vi "Single Cscan - DAQ Trigger.vi"(6 "Frequency":cluster{"Clock, kHz":dbl, "Freq, kHz":dbl}={"Clock, kHz"=920.0, "Freq, kHz"=46.0} {"Clock, kHz" format="%#_13g"}, 7 "# Extra":cluster{"# ARpt_extra":i32, "#Brtn_extra":i32}={"# ARpt_extra"=5, "#Brtn_extra"=40}, 9 "Galvo VPP":cluster{"VPP-X":dbl, "VPP-Y":dbl}={"VPP-X"=5.0, "VPP-Y"=5.0}, 10 "Scan Repeat":cluster{"# A rpt":i32, "# B rpt":i32}={"# A rpt"=1, "# B rpt"=1}, 11 "# Points":cluster{"# Aline":i32, "# B scan":i32}={"# Aline"=500, "# B scan"=500}) -> (2 "Galvo X&Trigger":waveform(dbl)[](graph)=[{"t0"=timestamp(0 s since 1904-01-01), "dt"=1.0, "Y"=array[3800 elements]}, {"t0"=timestamp(0 s since 1904-01-01), "dt"=1.0, "Y"=array[3800 elements]}])   [LabVIEW 2017]
uses:
  <vilib>/Waveform/WDTOps.llb/WDT Append Waveforms DBL.vi
  <vilib>/measure/NI_MABase.lvlib
panel:
  out "input cluster":cluster{"Fs":dbl, "#s":dbl}
  out "size(s)":i32
  out "#Brtn_extra":i32
  out "dVY":dbl
  out "# A Rpt Delay":i32
  out "# B rtn":i32
  out "# A repeat":i32
  out "dVX":dbl
  out "S/F":dbl
  out "VPP-Y":dbl
  out "VPP-X":dbl
  out "Clock, kHz":dbl
  out "Freq, kHz":dbl
  out "# A Total":i32
  out "# Aline":i32
  out "# B scan":i32
  out "# B Repeat":i32
  # "Single Cscan - DAQ Trigger"
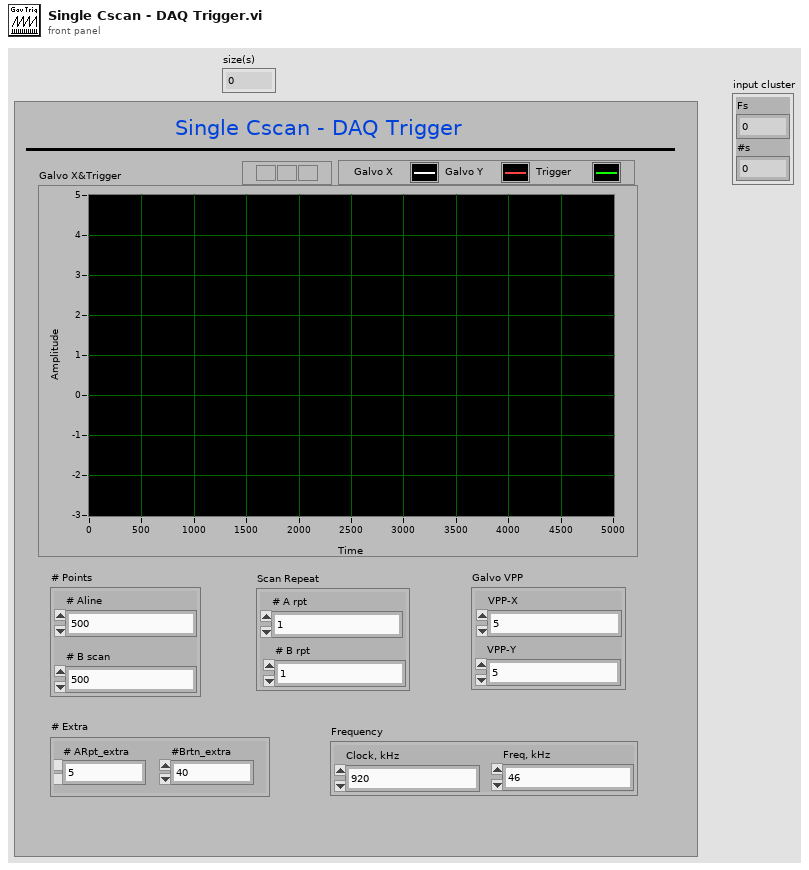
[diagram p1: front panel]
types:
  T1 = enum16{"Sine Wave", "Triangle Wave", "Square Wave", "Sawtooth Wave"}
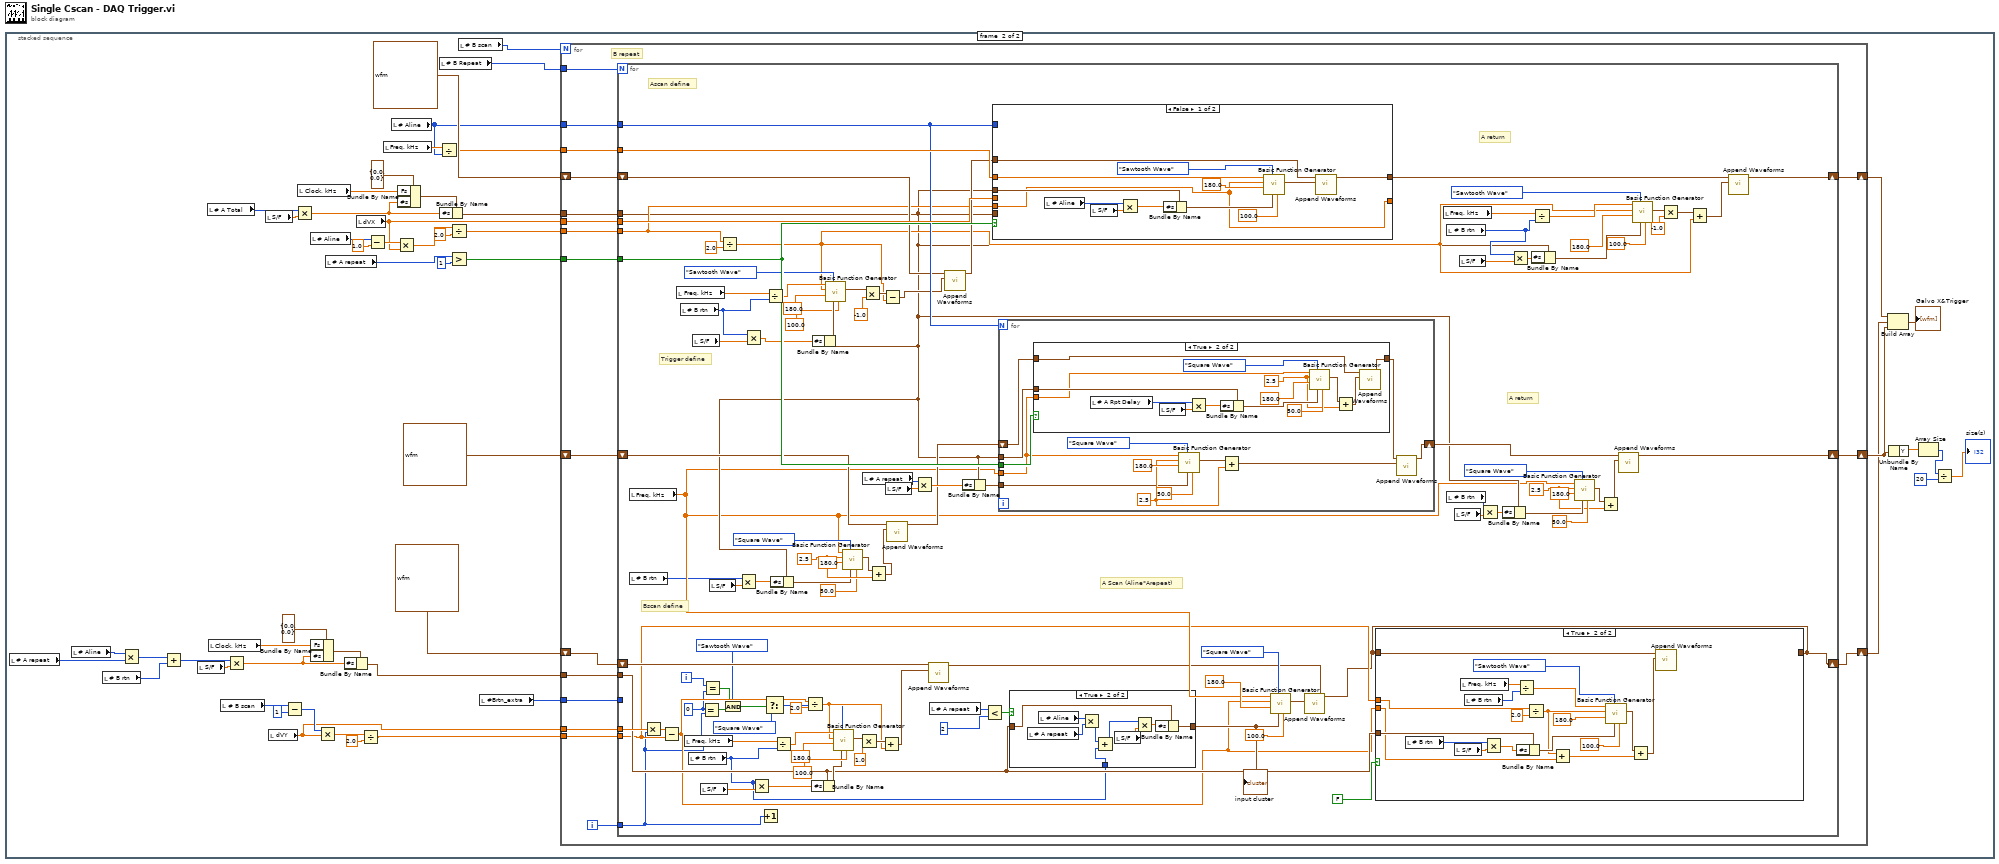
[diagram p0: block diagram]
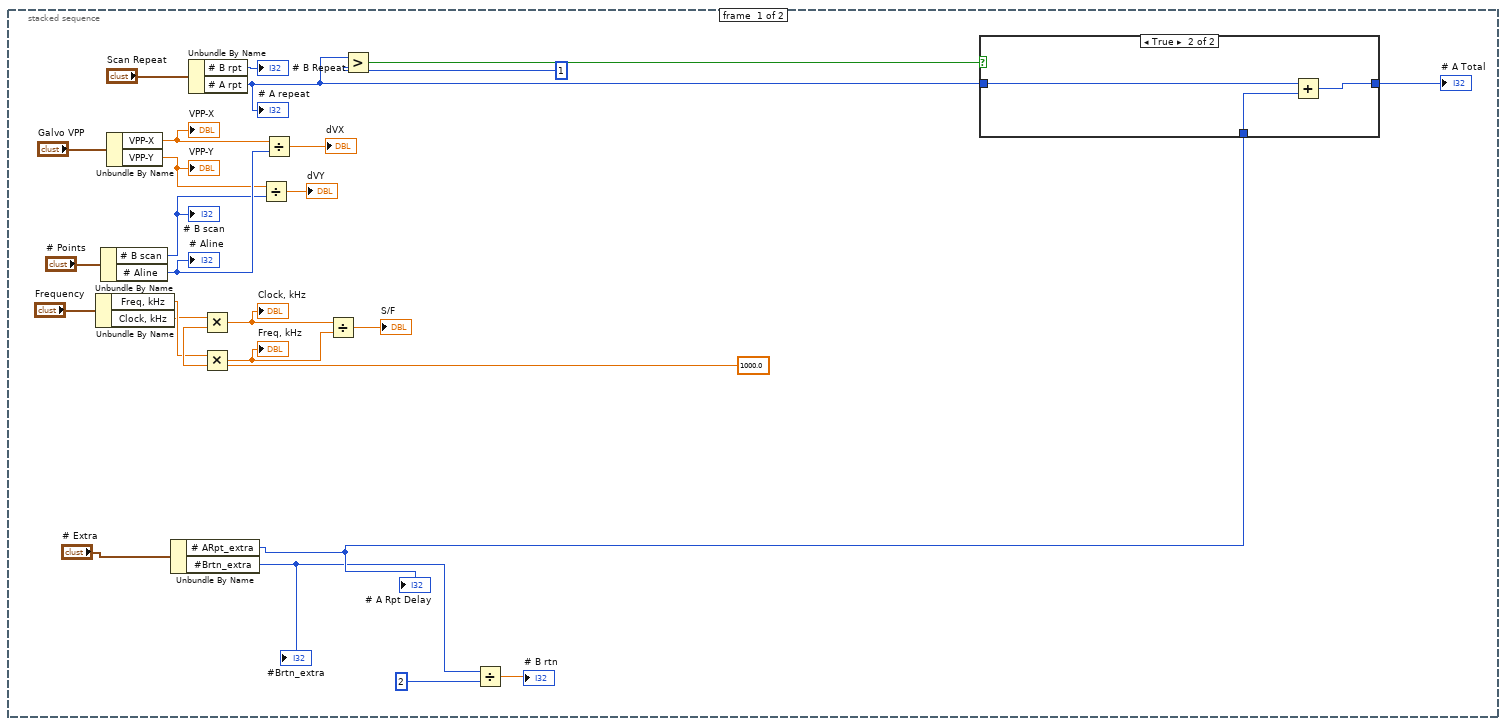
[diagram p2: hidden frame]
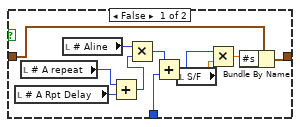
[diagram p4: hidden frame]
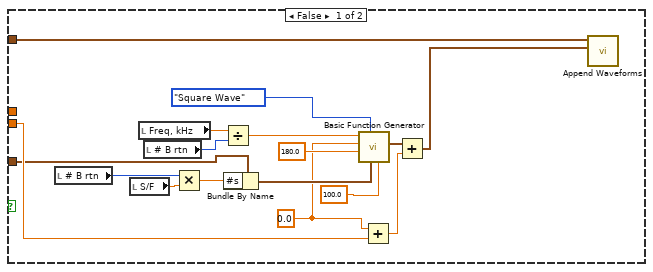
[diagram p5: hidden frame]
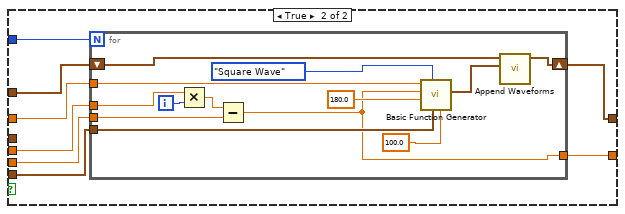
[diagram p7: hidden frame]
diagram:
  n1 = stacked-sequence {
    frame #0 {
      w26 = 1000.0 ("y")
      n2 = Unbundle By Name("Frequency") -> ("Freq, kHz"=w25:dbl, "Clock, kHz"=w21:dbl)
      n3 = Unbundle By Name("# Points") -> ("# B scan"=w2:i32, "# Aline"=w12:i32)
      "# B scan" <- w2
      "# Aline" <- w12
      n4 = Unbundle By Name("Galvo VPP") -> ("VPP-X"=w11:dbl, "VPP-Y"=w3:dbl)
      "VPP-X" <- w11
      "VPP-Y" <- w3
      n5 = Unbundle By Name("# Extra") -> ("# ARpt_extra"=w8:i32, "#Brtn_extra"=w7:i32)
      "# A Rpt Delay" <- w8
      "#Brtn_extra" <- w7
      n6 = Unbundle By Name("Scan Repeat") -> ("# B rpt"=→"# B Repeat":i32, "# A rpt"=w9:i32)
      "# A repeat" <- w9
      n7 = Multiply(x=w21, y=w26) -> (x*y=w15:dbl)
      "Clock, kHz" <- w15
      n8 = Multiply(x=w25, y=w26) -> (x*y=w14:dbl)
      "Freq, kHz" <- w14
      n9 = Divide(x=w3, y=w2) -> (x/y=→"dVY":dbl)
      n10 = Divide(x=w11, y=w12) -> (x/y=→"dVX":dbl)
      n11 = Divide(x=w15, y=w14) -> (x/y=→"S/F":dbl)
      n12 = Greater?(x=w9, y=1) -> (0:w22:bool)
      n13 = Divide(x=w7, y=2) -> (x/y=→"# B rtn":dbl)
      n14 = case shown="True" w22 {
        tunnel: w9 -> [w27 w30]
        tunnel: [w27 w29] -> w24
        tunnel: w8 -> [_ w28]
        frame False {
        }
        frame True {
          n15 = Add(x=w30, y=w28) -> (x+y=w29:i32)
        }
      }
      "# A Total" <- w24
    }
    frame #1 {
      n16 = local read "# A repeat"() -> (w48:i32)
      n17 = local read "# Aline"() -> (w49:i32)
      n18 = local read "# B rtn"() -> (w51:i32)
      n19 = Multiply(x=w49, y=w48) -> (x*y=w47:i32)
      n20 = Add(x=w47, y=w51) -> (x+y=w44:i32)
      n21 = local read "S/F"() -> (w45:dbl)
      n22 = local read "# A Total"() -> (w69:i32)
      n23 = local read "Clock, kHz"() -> (w46:dbl)
      n24 = local read "# B scan"() -> (w50:i32)
      n25 = Multiply(x=w44, y=w45) -> (x*y=w43:dbl)
      n26 = local read "S/F"() -> (w68:dbl)
      n27 = local read "dVY"() -> (w40:dbl)
      n28 = Subtract(x=w50, y=1) -> (x-y=w54:i32)
      n29 = Multiply(x=w69, y=w68) -> (x*y=w67:dbl)
      n30 = local read "Clock, kHz"() -> (w70:dbl)
      n31 = local read "# Aline"() -> (w71:i32)
      n32 = Bundle By Name(cluster=cluster{"Fs":dbl, "#s":dbl} {"Fs"=0.0, "#s"=0.0} ("input cluster"), "Fs"=w46, "#s"=w43) -> (w56:cluster{"Fs":dbl, "#s":dbl})
      n33 = Multiply(x=w54, y=w40) -> (x*y=w53:dbl)
      n34 = local read "# A repeat"() -> (w66:i32)
      n35 = Bundle By Name(cluster=w56, "#s"=w43) -> (w41:cluster{"Fs":dbl, "#s":dbl})
      n36 = local read "dVX"() -> (w60:dbl)
      n37 = Divide(x=w53, y=2.0) -> (x/y=w39:dbl)
      n38 = Subtract(x=w71, y=1.0) -> (x-y=w73:dbl)
      n39 = local read "Freq, kHz"() -> (w63:dbl)
      n40 = local read "# Aline"() -> (w62:i32)
      n41 = Multiply(x=w73, y=w60) -> (x*y=w77:dbl)
      n42 = Bundle By Name(cluster=cluster{"Fs":dbl, "#s":dbl} {"Fs"=0.0, "#s"=0.0} ("input cluster"), "Fs"=w70, "#s"=w67) -> (w78:cluster{"Fs":dbl, "#s":dbl})
      n43 = Divide(x=w63, y=w62) -> (x/y=w61:dbl)
      n44 = local read "# B Repeat"() -> (w72:i32)
      n45 = Bundle By Name(cluster=w78, "#s"=w67) -> (w80:cluster{"Fs":dbl, "#s":dbl})
      n46 = Divide(x=w77, y=2.0) -> (x/y=w75:dbl)
      n47 = Greater?(x=w66, y=1) -> (0:w64:bool)
      n48 = local read "# B scan"() -> (w38:i32)
      n49 = local read "#Brtn_extra"() -> (w37:i32)
      n50 = for {
        N: w38 -> [_]
        tunnel: w80 -> [w99]
        tunnel: w75 -> [w98]
        tunnel: w72 -> [w97]
        tunnel: w64 -> [w96]
        tunnel: w62 -> [w95]
        tunnel: w61 -> [w94]
        tunnel: w60 -> [w93]
        tunnel: w41 -> [w89]
        tunnel: w40 -> [w88]
        tunnel: w39 -> [w87]
        shift-right: [w91] -> w58
        shift-left: waveform(dbl) {"t0"=timestamp(0 s since 1904-01-01), "dt"=1.0, "Y"=[]} ("waveform out") -> [w100]
        shift-right: [w86] -> w36
        shift-left: waveform(dbl) {"t0"=timestamp(0 s since 1904-01-01), "dt"=1.0, "Y"=[]} ("waveform out") -> [w92]
        shift-right: [w85] -> w31
        shift-left: waveform(dbl) {"t0"=timestamp(0 s since 1904-01-01), "dt"=1.0, "Y"=[]} ("waveform out") -> [w90]
        tunnel: w37 -> [w84]
        i -> [w83]
        # "B repeat"
        n51 = for {
          N: w97 -> [_]
          tunnel: w95 -> [w183]
          tunnel: w93 -> [w207]
          tunnel: w99 -> [w145]
          tunnel: w98 -> [w167]
          shift-right: [w116] -> w91
          shift-left: w100 -> [w171]
          tunnel: w96 -> [w182]
          tunnel: w94 -> [w206]
          shift-right: [w115] -> w86
          shift-left: w92 -> [w149]
          tunnel: w89 -> [w128]
          tunnel: w88 -> [w137]
          tunnel: w87 -> [w125]
          shift-right: [w117] -> w85
          shift-left: w90 -> [w127]
          tunnel: w84 -> [_]
          tunnel: w83 -> [w113]
          i -> [w110]
          w109 = 0 ("x")
          w157 = 2.5 ("amplitude")
          w158 = 2.5 ("amplitude")
          # "Ascan define"
          # "Trigger define"
          # "Bscan define"
          # "A return"
          # "A Scan (Aline*Arepeat)"
          # "A return"
          n52 = local read "Freq, kHz"() -> (w138:dbl)
          n53 = local read "# B rtn"() -> (w136:i32)
          n54 = Multiply(x=w137, y=w113) -> (x*y=w142:dbl)
          n55 = Subtract(x=w142, y=w125) -> (x-y=w123:dbl)
          n56 = local read "Freq, kHz"() -> (w177:dbl)
          n57 = local read "# B rtn"() -> (w180:i32)
          n58 = local read "Freq, kHz"() -> (w131:dbl)
          n59 = local read "# B rtn"() -> (w103:i32)
          n60 = local read "S/F"() -> (w176:dbl)
          n61 = local read "S/F"() -> (w132:dbl)
          n62 = Equal?(x=w109, y=w113) -> (x = y?=w108:bool)
          n63 = Equal?(x=w110, y=w109) -> (x = y?=w107:bool)
          n64 = local read "S/F"() -> (w153:dbl)
          n65 = Divide(x=w167, y=2.0) -> (x/y=w161:dbl)
          n66 = And(x=w107, y=w108) -> (x .and. y?=w106:bool)
          n67 = Multiply(x=w136, y=w153) -> (x*y=w154:dbl)
          n68 = Multiply(x=w180, y=w176) -> (x*y=w179:dbl)
          n69 = Multiply(x=w103, y=w132) -> (x*y=w129:dbl)
          n70 = Increment(x=w113) -> ()  [unwired: 1 out]
          n71 = Select(t=T1."Sawtooth Wave" ("signal type"), s=w106, f=T1."Square Wave" ("signal type")) -> (s? t:f=w111:T1)
          n72 = Divide(x=w177, y=w180) -> (x/y=w178:dbl)
          n73 = Bundle By Name(cluster=w145, "#s"=w154) -> (w150:cluster{"Fs":dbl, "#s":dbl})
          n74 = Divide(x=w131, y=w103) -> (x/y=w130:dbl)
          n75 = Divide(x=w123, y=2.0) -> (x/y=w119:dbl)
          n76 = Bundle By Name(cluster=w128, "#s"=w129) -> (w133:cluster{"Fs":dbl, "#s":dbl})
          n77 = Bundle By Name(cluster=w145, "#s"=w179) -> (w175:cluster{"Fs":dbl, "#s":dbl})
          n78 = call <vilib>:"Basic Function Generator.vi"("square wave duty cycle (%)"=100.0, "sampling info"=w175, "signal type"=T1."Sawtooth Wave", "phase"=180.0, "amplitude"=w161, "frequency"=w178) -> ("signal out"=w169:waveform(dbl))  [unwired: 3 in, 2 out]
          n79 = call <vilib>:"Basic Function Generator.vi"("square wave duty cycle (%)"=100.0, "sampling info"=w133, "signal type"=w111, "phase"=180.0, "amplitude"=w119, "frequency"=w130) -> ("signal out"=w120:waveform(dbl))  [unwired: 3 in, 2 out]
          n80 = call <vilib>:"Basic Function Generator.vi"("square wave duty cycle (%)"=50.0, "sampling info"=w150, "signal type"=T1."Square Wave", "phase"=180.0, "amplitude"=w157, "frequency"=w138) -> ("signal out"=w155:waveform(dbl))  [unwired: 3 in, 2 out]
          n81 = Multiply(x=w120, y=1.0) -> (x*y=w121:waveform(dbl))
          n82 = Multiply(x=w169, y=-1.0) -> (x*y=w165:waveform(dbl))
          n83 = local read "# A repeat"() -> (w189:i32)
          n84 = Add(x=w155, y=w157) -> (x+y=w156:waveform(dbl))
          n85 = Add(x=w121, y=w119) -> (x+y=w105:waveform(dbl))
          n86 = Subtract(x=w165, y=w161) -> (x-y=w164:waveform(dbl))
          n87 = local read "S/F"() -> (w187:dbl)
          n88 = call-poly <vilib>:"Append Waveforms.vi"("waveform B"=w156, "waveform A"=w149) -> ("waveform out"=w148:waveform(dbl))  [unwired: 8 in, 1 out]
          n89 = Multiply(x=w189, y=w187) -> (x*y=w188:dbl)
          n90 = call-poly <vilib>:"Append Waveforms.vi"("waveform B"=w105, "waveform A"=w127) -> ("waveform out"=w126:waveform(dbl))  [unwired: 8 in, 1 out]
          n91 = local read "# A repeat"() -> (w140:i32)
          n92 = call-poly <vilib>:"Append Waveforms.vi"("waveform B"=w164, "waveform A"=w171) -> ("waveform out"=w170:waveform(dbl))  [unwired: 8 in, 1 out]
          n93 = Bundle By Name(cluster=w145, "#s"=w188) -> (w192:cluster{"Fs":dbl, "#s":dbl})
          n94 = Less?(x=w140, y=2) -> (x < y?=w101:bool)
          n95 = case shown="False" w182 {
            tunnel: w170 -> [w293 w312]
            tunnel: w183 -> [_ w311]
            tunnel: w207 -> [_ w310]
            tunnel: w145 -> [_ w309]
            tunnel: w167 -> [w292 w308]
            tunnel: [w294 w307] -> w199
            tunnel: [w292 w306] -> _
            tunnel: w206 -> [w301 w305]
            tunnel: w145 -> [w299 _]
            frame False {
              n96 = local read "# Aline"() -> (w298:i32)
              n97 = local read "S/F"() -> (w297:dbl)
              n98 = Multiply(x=w298, y=w297) -> (x*y=w296:dbl)
              n99 = Bundle By Name(cluster=w299, "#s"=w296) -> (w300:cluster{"Fs":dbl, "#s":dbl})
              n100 = call <vilib>:"Basic Function Generator.vi"("square wave duty cycle (%)"=100.0, "sampling info"=w300, "signal type"=T1."Sawtooth Wave", "phase"=180.0, "amplitude"=w292, "frequency"=w301) -> ("signal out"=w295:waveform(dbl))  [unwired: 3 in, 2 out]
              n101 = call-poly <vilib>:"Append Waveforms.vi"("waveform B"=w295, "waveform A"=w293) -> ("waveform out"=w294:waveform(dbl))  [unwired: 8 in, 1 out]
            }
            frame True {
              n102 = for {
                N: w311 -> [_]
                tunnel: w305 -> [w319]
                tunnel: w309 -> [w323]
                tunnel: w310 -> [w321]
                shift-right: [w318] -> w307
                shift-left: w312 -> [w317]
                tunnel: w308 -> [w315]
                tunnel: [w314] -> w306
                i -> [w320]
                n103 = Multiply(x=w321, y=w320) -> (x*y=w316:dbl)
                n104 = Subtract(x=w316, y=w315) -> (x-y=w314:dbl)
                n105 = call <vilib>:"Basic Function Generator.vi"("square wave duty cycle (%)"=100.0, "sampling info"=w323, "signal type"=T1."Square Wave" ("signal type B"), "phase"=180.0, "amplitude"=w314, "frequency"=w319) -> ("signal out"=w324:waveform(dbl))  [unwired: 3 in, 2 out]
                n106 = call-poly <vilib>:"Append Waveforms.vi"("waveform B"=w324, "waveform A"=w317) -> ("waveform out"=w318:waveform(dbl))  [unwired: 8 in, 1 out]
              }
            }
          }
          n107 = for {
            N: w183 -> [_]
            tunnel: w192 -> [w269]
            tunnel: w145 -> [w268]
            tunnel: w182 -> [w267]
            tunnel: w138 -> [w266]
            shift-right: [w276] -> w194
            shift-left: w148 -> [w264]
            w270 = 2.5 ("amplitude")
            n108 = case shown="True" w267 {
              tunnel: w268 -> [_ w289]
              tunnel: w266 -> [_ w287]
              tunnel: [w277 w282] -> w265
              tunnel: w264 -> [w277 w283]
              frame False {
              }
              frame True {
                w278 = 2.5 ("amplitude")
                n109 = local read "# A Rpt Delay"() -> (w284:i32)
                n110 = local read "S/F"() -> (w285:dbl)
                n111 = Multiply(x=w284, y=w285) -> (x*y=w291:dbl)
                n112 = Bundle By Name(cluster=w289, "#s"=w291) -> (w290:cluster{"Fs":dbl, "#s":dbl})
                n113 = call <vilib>:"Basic Function Generator.vi"("square wave duty cycle (%)"=50.0, "sampling info"=w290, "signal type"=T1."Square Wave", "phase"=180.0, "amplitude"=w278, "frequency"=w287) -> ("signal out"=w281:waveform(dbl))  [unwired: 3 in, 2 out]
                n114 = Add(x=w281, y=w278) -> (x+y=w279:waveform(dbl))
                n115 = call-poly <vilib>:"Append Waveforms.vi"("waveform B"=w279, "waveform A"=w283) -> ("waveform out"=w282:waveform(dbl))  [unwired: 8 in, 1 out]
              }
            }
            n116 = call <vilib>:"Basic Function Generator.vi"("square wave duty cycle (%)"=50.0, "sampling info"=w269, "signal type"=T1."Square Wave" ("signal type B"), "phase"=180.0, "amplitude"=w270, "frequency"=w266) -> ("signal out"=w272:waveform(dbl))  [unwired: 3 in, 2 out]
            n117 = Add(x=w272, y=w270) -> (x+y=w271:waveform(dbl))
            n118 = call-poly <vilib>:"Append Waveforms.vi"("waveform B"=w271, "waveform A"=w265) -> ("waveform out"=w276:waveform(dbl))  [unwired: 8 in, 1 out]
          }
          n119 = case shown="True" w101 {
            tunnel: w128 -> [w215 w227]
            tunnel: [w214 w226] -> w139
            tunnel: w103 -> [w211 w220]
            frame False {
              n120 = local read "# A Rpt Delay"() -> (w210:i32)
              n121 = local read "# A repeat"() -> (w209:i32)
              n122 = local read "# Aline"() -> (w218:i32)
              n123 = Add(x=w209, y=w210) -> (x+y=w208:i32)
              n124 = Multiply(x=w218, y=w208) -> (x*y=w213:i32)
              n125 = Add(x=w213, y=w211) -> (x+y=w212:i32)
              n126 = local read "S/F"() -> (w217:dbl)
              n127 = Multiply(x=w212, y=w217) -> (x*y=w216:dbl)
              n128 = Bundle By Name(cluster=w215, "#s"=w216) -> (w214:cluster{"Fs":dbl, "#s":dbl})
            }
            frame True {
              n129 = local read "# A repeat"() -> (w224:i32)
              n130 = local read "# Aline"() -> (w225:i32)
              n131 = Multiply(x=w225, y=w224) -> (x*y=w221:i32)
              n132 = Add(x=w221, y=w220) -> (x+y=w219:i32)
              n133 = local read "S/F"() -> (w223:dbl)
              n134 = Multiply(x=w219, y=w223) -> (x*y=w222:dbl)
              n135 = Bundle By Name(cluster=w227, "#s"=w222) -> (w226:cluster{"Fs":dbl, "#s":dbl})
            }
          }
          "input cluster" <- w139
          n136 = call <vilib>:"Basic Function Generator.vi"("square wave duty cycle (%)"=100.0, "sampling info"=w139, "signal type"=T1."Square Wave" ("signal type B"), "phase"=180.0, "amplitude"=w123, "frequency"=w138) -> ("signal out"=w104:waveform(dbl))  [unwired: 3 in, 2 out]
          n137 = call-poly <vilib>:"Append Waveforms.vi"("waveform B"=w104, "waveform A"=w126) -> ("waveform out"=w117:waveform(dbl))  [unwired: 8 in, 1 out]
          n138 = case shown="True" FALSE {
            tunnel: w117 -> [w231 w253]
            tunnel: w117 -> [_ _]
            tunnel: w123 -> [w230 w246]
            tunnel: w125 -> [_ w251]
            tunnel: w128 -> [w229 w252]
            frame False {
              w228 = 0.0 ("y")
              n139 = local read "# B rtn"() -> (w240:i32)
              n140 = local read "S/F"() -> (w239:dbl)
              n141 = local read "Freq, kHz"() -> (w237:dbl)
              n142 = local read "# B rtn"() -> (w236:i32)
              n143 = Multiply(x=w240, y=w239) -> (x*y=w238:dbl)
              n144 = Divide(x=w237, y=w236) -> (x/y=w235:dbl)
              n145 = Bundle By Name(cluster=w229, "#s"=w238) -> (w241:cluster{"Fs":dbl, "#s":dbl})
              n146 = call <vilib>:"Basic Function Generator.vi"("square wave duty cycle (%)"=100.0, "sampling info"=w241, "signal type"=T1."Square Wave", "phase"=180.0, "amplitude"=w228, "frequency"=w235) -> ("signal out"=w234:waveform(dbl))  [unwired: 3 in, 2 out]
              n147 = Add(x=w228, y=w230) -> (x+y=w232:dbl)
              n148 = Add(x=w234, y=w232) -> (x+y=w233:waveform(dbl))
              n149 = call-poly <vilib>:"Append Waveforms.vi"("waveform B"=w233, "waveform A"=w231) -> ()  [unwired: 8 in, 2 out]
            }
            frame True {
              n150 = local read "# B rtn"() -> (w259:i32)
              n151 = local read "S/F"() -> (w258:dbl)
              n152 = local read "Freq, kHz"() -> (w256:dbl)
              n153 = local read "# B rtn"() -> (w255:i32)
              n154 = Multiply(x=w259, y=w258) -> (x*y=w257:dbl)
              n155 = Divide(x=w256, y=w255) -> (x/y=w254:dbl)
              n156 = Bundle By Name(cluster=w252, "#s"=w257) -> (w260:cluster{"Fs":dbl, "#s":dbl})
              n157 = Divide(x=w251, y=2.0) -> (x/y=w245:dbl)
              n158 = Add(x=w245, y=w246) -> (x+y=w247:dbl)
              n159 = call <vilib>:"Basic Function Generator.vi"("square wave duty cycle (%)"=100.0, "sampling info"=w260, "signal type"=T1."Sawtooth Wave", "phase"=180.0, "amplitude"=w245, "frequency"=w254) -> ("signal out"=w249:waveform(dbl))  [unwired: 3 in, 2 out]
              n160 = Add(x=w249, y=w247) -> (x+y=w248:waveform(dbl))
              n161 = call-poly <vilib>:"Append Waveforms.vi"("waveform B"=w248, "waveform A"=w253) -> ()  [unwired: 8 in, 2 out]
            }
          }
          n162 = local read "Freq, kHz"() -> (w198:dbl)
          n163 = local read "# B rtn"() -> (w181:i32)
          n164 = local read "# B rtn"() -> (w186:i32)
          n165 = local read "S/F"() -> (w185:dbl)
          n166 = local read "S/F"() -> (w201:dbl)
          n167 = Multiply(x=w186, y=w185) -> (x*y=w184:dbl)
          n168 = Bundle By Name(cluster=w145, "#s"=w184) -> (w193:cluster{"Fs":dbl, "#s":dbl})
          n169 = Multiply(x=w181, y=w201) -> (x*y=w196:dbl)
          n170 = Divide(x=w198, y=w181) -> (x/y=w197:dbl)
          n171 = Bundle By Name(cluster=w145, "#s"=w196) -> (w202:cluster{"Fs":dbl, "#s":dbl})
          n172 = call <vilib>:"Basic Function Generator.vi"("square wave duty cycle (%)"=50.0, "sampling info"=w193, "signal type"=T1."Square Wave", "phase"=180.0, "amplitude"=w158, "frequency"=w138) -> ("signal out"=w160:waveform(dbl))  [unwired: 3 in, 2 out]
          n173 = Add(x=w160, y=w158) -> (x+y=w159:waveform(dbl))
          n174 = call-poly <vilib>:"Append Waveforms.vi"("waveform B"=w159, "waveform A"=w194) -> ("waveform out"=w115:waveform(dbl))  [unwired: 8 in, 1 out]
          n175 = call <vilib>:"Basic Function Generator.vi"("square wave duty cycle (%)"=100.0, "sampling info"=w202, "signal type"=T1."Sawtooth Wave", "phase"=180.0, "amplitude"=w161, "frequency"=w197) -> ("signal out"=w195:waveform(dbl))  [unwired: 3 in, 2 out]
          n176 = Multiply(x=w195, y=-1.0) -> (x*y=w163:waveform(dbl))
          n177 = Add(x=w163, y=w161) -> (x+y=w162:waveform(dbl))
          n178 = call-poly <vilib>:"Append Waveforms.vi"("waveform B"=w162, "waveform A"=w199) -> ("waveform out"=w116:waveform(dbl))  [unwired: 8 in, 1 out]
        }
      }
      n179 = Build Array(w58, w31, w36) -> (→"Galvo X&Trigger":waveform(dbl)[])
      n180 = Unbundle By Name(w36) -> ("Y"=w35:dbl[])
      n181 = Array Size(array=w35) -> (size(s)=w34:i32)
      n182 = Divide(x=w34, y=20) -> (x/y=→"size(s)":dbl)
    }
  }
